vi "Errosion_number.vi"(2 "Loop number":i32, 3 "Insect-data-array":dbl[][](array[numeric])) -> (0 "Length of largest insect from latest computer vision picture":dbl, 1 "Errosion number":i32)   [LabVIEW 2022 SP3]
doc: "Determines a sutable number of errosions to apply to the computer vision based on the largest insect found in the last computer vision image"
panel:
  out "Length of 6. insect ore 1. in case of less than 6 insects":dbl
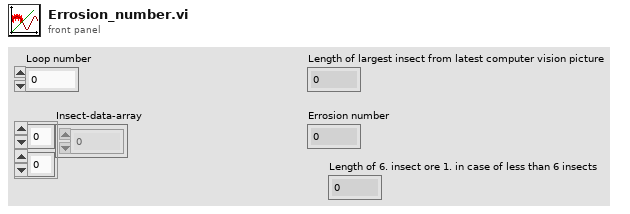
[diagram p1: front panel]
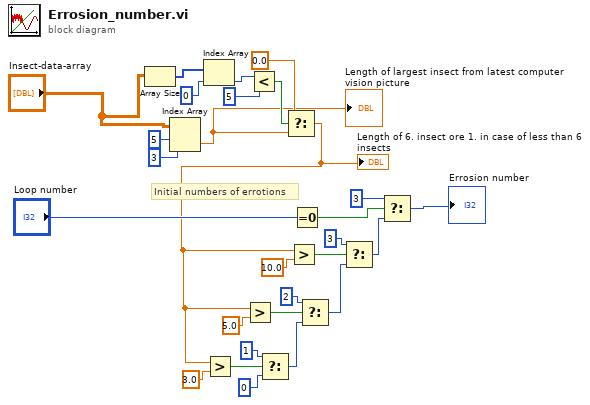
[diagram p0: block diagram]
diagram:
  # "Initial numbers of errotions"
  n1 = Array Size(array="Insect-data-array") -> (size(s)=w8:i32[])
  n2 = Index Array(array="Insect-data-array", index (row)=5, index (col)=3 ("disabled index (col)")) -> (element=w2:dbl)
  "Length of largest insect from latest computer vision picture" <- w2
  n3 = Index Array(array=w8, index=0) -> (element=w6:i32)
  n4 = Less?(x=w6, y=5) -> (x < y?=w5:bool)
  n5 = Select(t=0.0, s=w5, f=w2) -> (s? t:f=w3:dbl)
  "Length of 6. insect ore 1. in case of less than 6 insects" <- w3
  n6 = Greater?(x=w3, y=3.0) -> (0:w22:bool)
  n7 = Greater?(x=w3, y=5.0) -> (0:w21:bool)
  n8 = Select(t=1, s=w22, f=0) -> (s? t:f=w25:i32)
  n9 = Greater?(x=w3, y=10.0) -> (0:w16:bool)
  n10 = Equal To 0?(x="Loop number") -> (x = 0?=w13:bool)
  n11 = Select(t=2, s=w21, f=w25) -> (s? t:f=w24:i32)
  n12 = Select(t=3, s=w16, f=w24) -> (s? t:f=w17:i32)
  n13 = Select(t=3, s=w13, f=w17) -> (s? t:f=→"Errosion number":i32)
